vi "edit.vi"(8 "error in (no error)":errorcluster, 11 "BaseSetting in":refnum<class "ProcessSettings.lvclass">) -> (0 "error out":errorcluster, 2 "cancelIsTrue out":bool, 3 "BaseSetting out":refnum<class "ProcessSettings.lvclass">)   [LabVIEW 2016, in "Settings.lvlib" / "ProcessSettings.lvclass"]
uses:
  ProcessSettings.lvclass
  C:/Users/aanania/Documents/ts_monochromator_windows/WindowsController/MonoSettings/Settings/Settings/Setting.lvclass
  ConfigurationTypedefs/Base/TCPConfiguration.ctl
  ConfigurationTypedefs/Base/MonochromatorSettings.ctl
  Typedefs/wavelength.ctl
  Typedefs/slitWidth.ctl
  Settings/Setting.lvclass/Setting.ctl
  <vilib>/Utility/xml.llb/Write to XML File(string).vi
  Settings/Setting.lvclass
  ConfigurationTypedefs/ConfigurationTypedefs.lvlib
panel:
  in  "SettingTab":enum32{"Monochromator Settings", "TCP Settings"}(tab)
  in  "MonoSettings":T1={"Force Init"=FALSE, "WavelengthMin"=300.0, "WavelengthMax"=0.0, "SlitWidthMin"=0.0, "SlitWidthMax"=0.0, "timeout"=600.0}
  in  "TCPConfiguration":T4={"IP"="127.0.0.1", "port_low"=50000, "port_up"=50000, "connection_timeout "=10, "reading_timeout"=10, "writing_timeout"=10}
  in  "cancelIsTrue":bool
  out "String":string
  in  "saveIsTrue":bool
  in  "Listbox":i32(listbox)
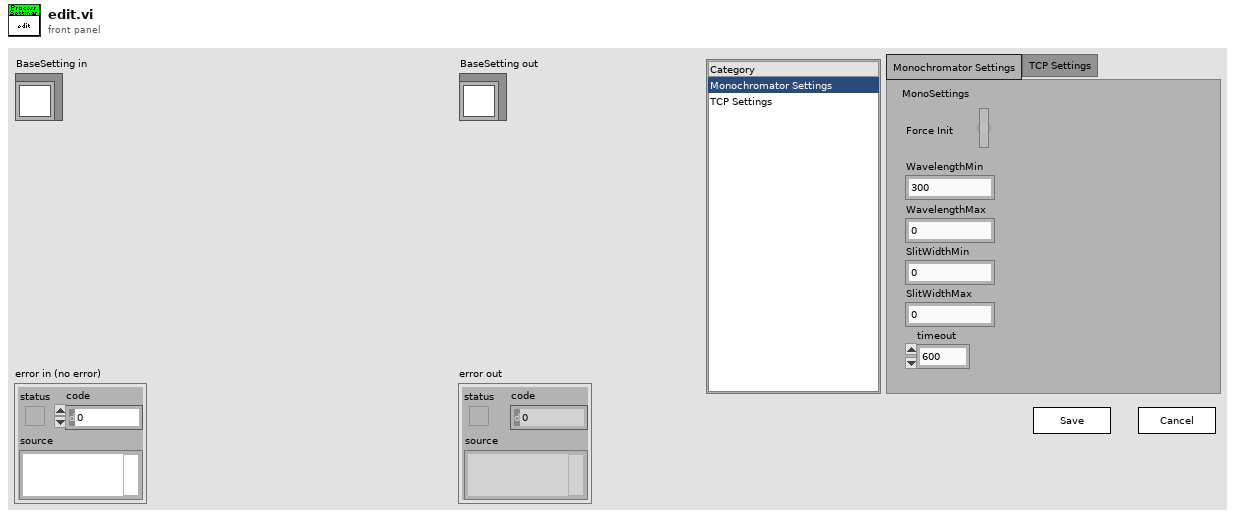
[diagram p1: front panel]
types:
  T1 = typedef "Settings.lvlib/ConfigurationTypedefs.lvlib/MonochromatorSettings.ctl" = cluster{"Force Init":bool, "WavelengthMin":T2, "WavelengthMax":T2, "SlitWidthMin":T3, "SlitWidthMax":T3, "timeout":dbl}
  T2 = typedef "wavelength.ctl" = dbl
  T3 = typedef "slitWidth.ctl" = dbl
  T4 = typedef "Settings.lvlib/ConfigurationTypedefs.lvlib/TCPConfiguration.ctl" = cluster{"IP":string, "port_low":u16, "port_up":u16, "connection_timeout ":i32, "reading_timeout":i32, "writing_timeout":i32}
  T5 = enum16{"open", "replace", "create", "open or create", "replace or create", "replace or create with confirmation"}
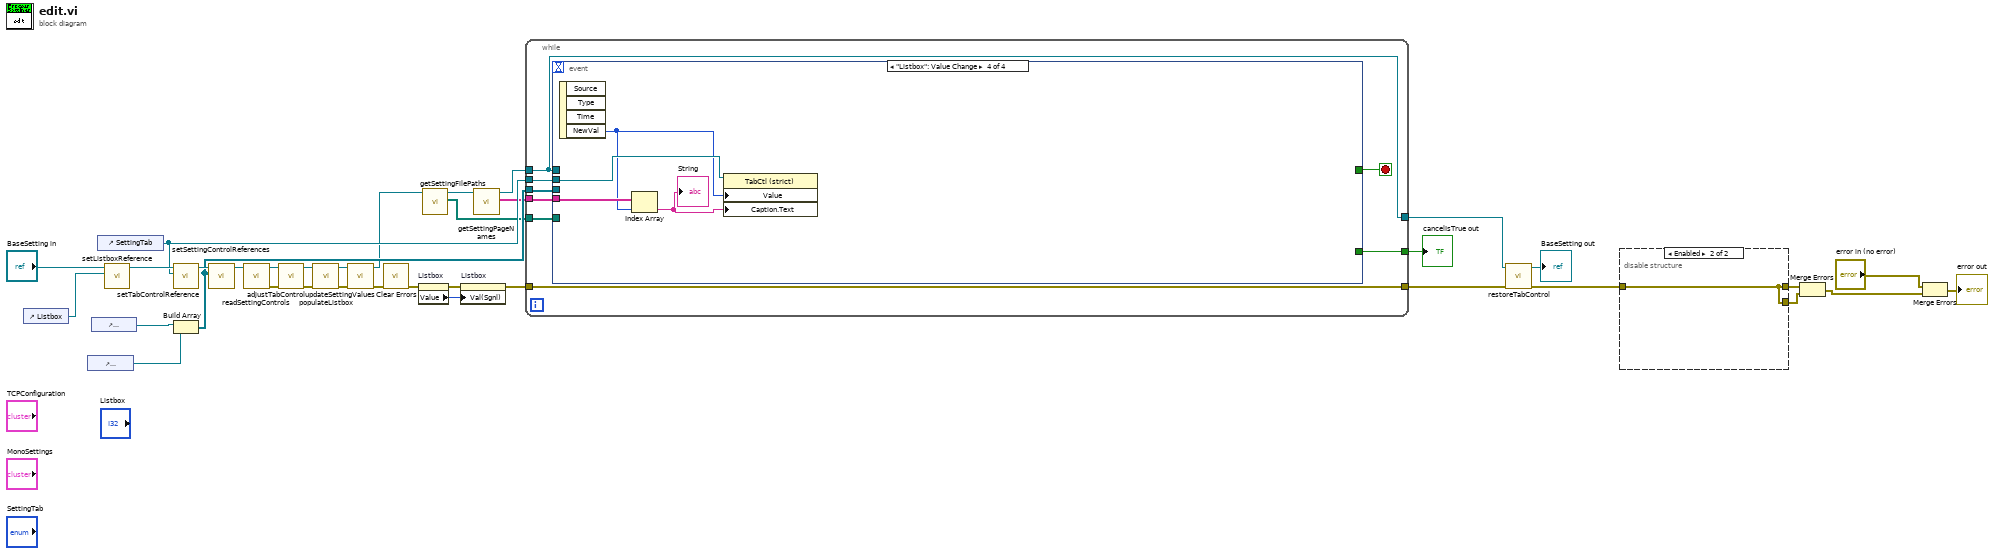
[diagram p0: block diagram]
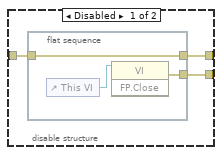
[diagram p2: hidden frame]
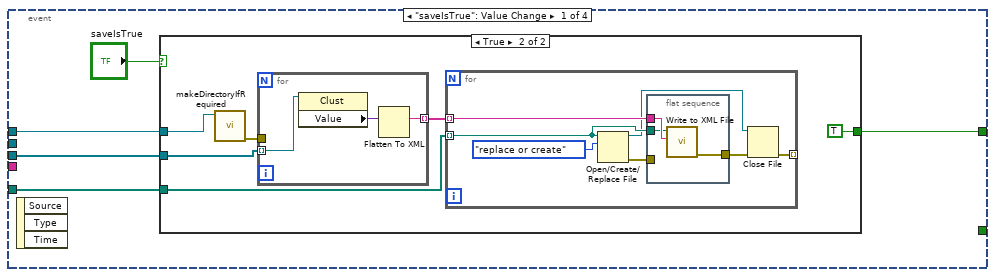
[diagram p3: hidden frame]
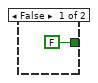
[diagram p4: hidden frame]
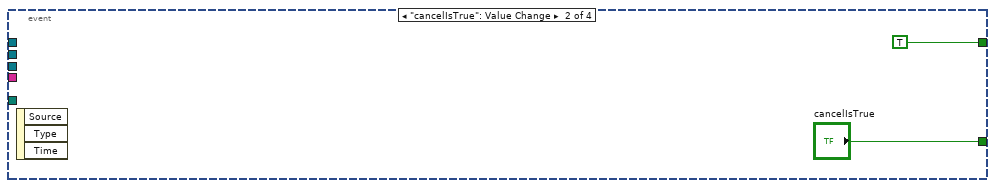
[diagram p5: hidden frame]
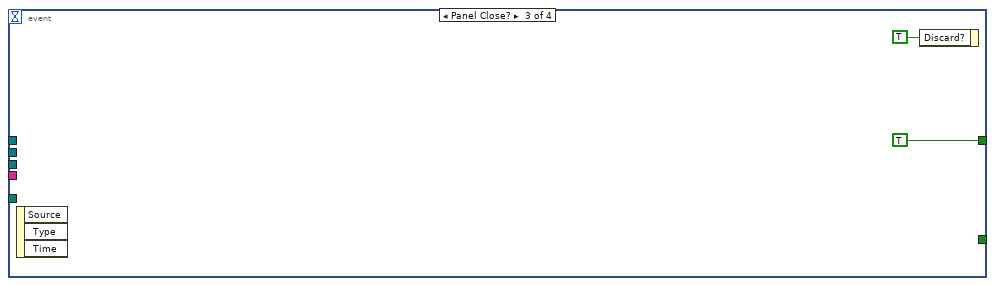
[diagram p6: hidden frame]
diagram:
  n1 = control-ref of="Listbox"() -> (w26:refnum<vi>)
  n2 = control-ref of="MonoSettings"() -> (w1:refnum<vi>)
  n3 = control-ref of="TCPConfiguration"() -> (w2:refnum<vi>)
  n4 = control-ref of="SettingTab"() -> (w23:refnum<vi>)
  n5 = call "setListboxReference.vi"("ListboxReference"=w26, "Setting in"="BaseSetting in") -> ("Setting out"=w25:refnum<class "ProcessSettings.lvclass">)  [unwired: 9 in]
  n6 = call "setTabControlReference.vi"("TabControlReference"=w23, "Setting in"=w25) -> ("Setting out"=w24:refnum<class "ProcessSettings.lvclass">)  [unwired: 9 in]
  n7 = Build Array(w2, w1) -> (w22:refnum<vi>[])
  n8 = call "setSettingControlReferences.vi"("SettingControlReferences"=w22, "Setting in"=w24) -> ("Setting out"=w17:refnum<class "ProcessSettings.lvclass">)  [unwired: 9 in]
  n9 = call "readSettingControls.vi"("BaseSetting in"=w17) -> ("error out"=w12:errorcluster, "BaseSetting out"=w16:refnum<class "ProcessSettings.lvclass">)  [unwired: 9 in]
  n10 = call "adjustTabControl.vi"("error in (no error)"=w12, "BaseSetting in"=w16) -> ("error out"=w11:errorcluster, "BaseSetting out"=w15:refnum<class "ProcessSettings.lvclass">)  [unwired: 8 in]
  n11 = call "populateListbox.vi"("error in (no error)"=w11, "BaseSetting in"=w15) -> ("error out"=w10:errorcluster, "BaseSetting out"=w14:refnum<class "ProcessSettings.lvclass">)  [unwired: 8 in]
  n12 = call "updateSettingValues.vi"("error in (no error)"=w10, "BaseSetting in"=w14) -> ("error out"=w5:errorcluster, "BaseSetting out"=w13:refnum<class "ProcessSettings.lvclass">)  [unwired: 8 in]
  n13 = call <vilib>:"Clear Errors.vi"("error in (no error)"=w5) -> ("error out"=w4:errorcluster)  [unwired: 5 in, 1 out]
  n14 = property on="Listbox" class="LstBox (strict)"(error in=w4) -> (error out=w34:errorcluster, "Value"=w35:i32)  [unwired: 1 in, 1 out]
  n15 = call "getSettingFilePaths.vi"("Setting in"=w13) -> ("SettingFilePaths"=w19:path[], "Setting out"=w21:refnum<class "ProcessSettings.lvclass">)  [unwired: 9 in]
  n16 = property on="Listbox" class="LstBox (strict)"(error in=w34, "Val(Sgnl)"=w35) -> (error out=w27:errorcluster)  [unwired: 1 in, 1 out]
  n17 = call "getSettingPageNames.vi"("Setting in"=w21) -> ("SettingPageNames"=w20:string[], "Setting out"=w18:refnum<class "ProcessSettings.lvclass">)  [unwired: 9 in]
  n18 = while {
    tunnel: w19 -> [w43]
    tunnel: w20 -> [w42]
    tunnel: w23 -> [w39]
    tunnel: w22 -> [w41]
    tunnel: [w36] -> w9
    tunnel: w18 -> [w36]
    tunnel: w27 -> [w38]
    tunnel: [w38] -> w6
    tunnel: [w37] -> w28
    stop <- w40 stop-if-true
    n19 = event shown="[3] \"Listbox\": Value Change" {
      selector: _ -> [_ _ _ _]
      dyn-events: _ -> [_ _ _ _]
      timeout: _ -> [_ _ _ _]
      tunnel: [w44 TRUE TRUE _] -> w40
      tunnel: w43 -> [w48 _ _ _]
      tunnel: w42 -> [_ _ _ w75]
      tunnel: w39 -> [_ _ _ w76]
      tunnel: w41 -> [w47 _ _ _]
      tunnel: [_ "cancelIsTrue" _ _] -> w37
      tunnel: w36 -> [w46 _ _ _]
      event "saveIsTrue": Value Change {
        n20 = event-data() -> ()  [unwired: 1 in, 3 out]
        n21 = case shown="True" "saveIsTrue" {
          tunnel: w48 -> [_ w55]
          tunnel: w47 -> [_ w54]
          tunnel: w46 -> [_ w51]
          tunnel: [FALSE TRUE] -> w44
          frame False {
          }
          frame True {
            n22 = call "makeDirectoryIfRequired.vi"("BaseSetting in"=w51) -> ("error out"=w50:errorcluster)  [unwired: 9 in, 1 out]
            n23 = for {
              tunnel: w54 -> [w68] mode=indexing
              tunnel: [w66] -> w53 mode=indexing
              tunnel: w50 -> [_]
              n24 = property class="Clust"(reference=w68) -> ("Value"=w67:variant)  [unwired: 1 in, 2 out]
              n25 = Flatten To XML(anything=w67) -> (xml string=w66:string)
            }
            n26 = for {
              tunnel: w55 -> [w59] mode=indexing
              tunnel: w53 -> [w62] mode=indexing
              tunnel: [w56] -> _ mode=indexing
              n27 = Open/Create/Replace File(file path (use dialog)=w59, operation (0:open)=T5."replace or create") -> (refnum out=w58:refnum<file>, error out=w60:errorcluster)  [unwired: 4 in, 1 out]
              n28 = flat-sequence {
                tunnel: w62 -> [w65]
                tunnel: [w64] -> w57
                tunnel: w60 -> [_]
                tunnel: w59 -> [w63]
                frame #0 {
                  n29 = call-poly <vilib>:"Write to XML File.vi"("XML Input"=w65, "XML File Path"=w63) -> ("error out"=w64:errorcluster)  [unwired: 7 in, 2 out]
                }
              }
              n30 = Close File(refnum=w58, error in=w57) -> (error out=w56:errorcluster)  [unwired: 1 out]
            }
          }
        }
      }
      event "cancelIsTrue": Value Change {
        n31 = event-data() -> ()  [unwired: 1 in, 3 out]
      }
      event Panel Close? {
        n32 = event-data() -> ()  [unwired: 1 in, 3 out]
        n33 = event-data("Discard?"=TRUE) -> ()  [unwired: 1 in, 1 out]
      }
      event "Listbox": Value Change {
        n34 = event-data() -> ("NewVal"=w74:i32)  [unwired: 1 in, 3 out]
        n35 = Index Array(array=w75, index=w74) -> (element=w73:string)
        "String" <- w73
        n36 = property class="TabCtl (strict)"(reference=w76, "Value"=w74, "Caption.Text"=w73) -> ()  [unwired: 1 in, 2 out]
      }
    }
  }
  "cancelIsTrue out" <- w28
  n37 = call "restoreTabControl.vi"("error in (no error)"=w6, "BaseSetting in"=w9) -> ("error out"=w7:errorcluster, "BaseSetting out"=→"BaseSetting out":refnum<class "ProcessSettings.lvclass">)  [unwired: 8 in]
  n38 = disable-structure shown="Enabled" {
    disable-tunnel: [w79 w83] -> w31
    disable-tunnel: [w78 w83] -> w29
    disable-tunnel: w7 -> [w77 w83]
    frame Disabled {
      n39 = flat-sequence {
        tunnel: [w81] -> w79
        tunnel: [w80] -> w78
        tunnel: w77 -> [w80]
        frame #0 {
          n40 = control-ref of="This VI"() -> (w82:refnum<vi>)
          n41 = invoke class="VI" method="FP.Close"(reference=w82) -> (error out=w81:errorcluster)  [unwired: 2 in, 2 out]
        }
      }
    }
    frame Enabled {
    }
  }
  n42 = Merge Errors(w29, w31) -> (w30:errorcluster)
  n43 = Merge Errors("error in (no error)", w30) -> (→"error out":errorcluster)
